vi "FrequencyAtEachBin (SubVI).vi"(9 "Rate of Measurement (Hz)":dbl, 10 "Length of Full FFT":i32, 11 "Length of Positive Half of FFT":dbl) -> (3 "Frequency Array":dbl[](array[numeric]))   [LabVIEW 2015]
uses:
  <vilib>/Analysis/1siggen.llb/Ramp Pattern by Delta.vi
  <vilib>/Analysis/NI_AALBase.lvlib
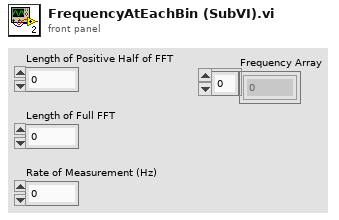
[diagram p1: front panel]
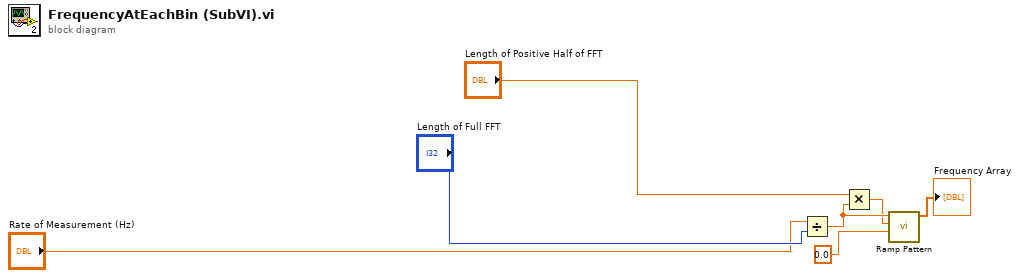
[diagram p0: block diagram]
diagram:
  n1 = Divide(x="Rate of Measurement (Hz)", y="Length of Full FFT") -> (x/y=w3:dbl)
  n2 = Multiply(x="Length of Positive Half of FFT", y=w3) -> (x*y=w2:dbl)
  n3 = call-poly <vilib>:"Ramp Pattern.vi"("start"=0.0, "end"=w2, "delta"=w3) -> ("Ramp Pattern"=→"Frequency Array":dbl[])  [unwired: 6 in, 2 out]
